vi "PV MiniTest Calibration.vi"(0 "VISA session":refnum<visa-resource-name>, 1 "Adress of unit":u16=1 min=1 max=999 step=1, 5 "Parameter":u16(ring) items=[" State of Calibration (read only)", " Calibration factor (read only)", " Start Calibration (write only)"], 11 "error in (no error)":errorcluster) -> (4 "dup VISA session":refnum<visa-resource-name>, 6 "response (data)":string, 15 "error out":errorcluster)   [LabVIEW 2021, in "Pfeiffer Vacuum.lvlib"]
doc: "There are 3 parameters available, only one of which can be enabled at a time. \n\n0 - Calibration State (default) - Para 667\n1 - Calibration factor (read only) - Para 696\n7 - Start Calibration (write only) - Para 699"
uses:
  <instrlib>/Pfeiffer Vacuum/Pfeiffer Vacuum.lvlib
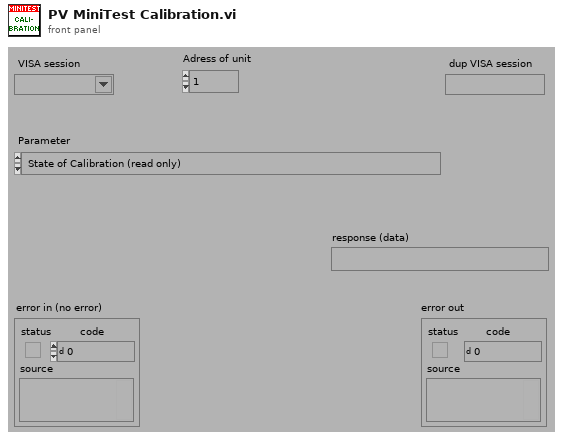
[diagram p1: front panel]
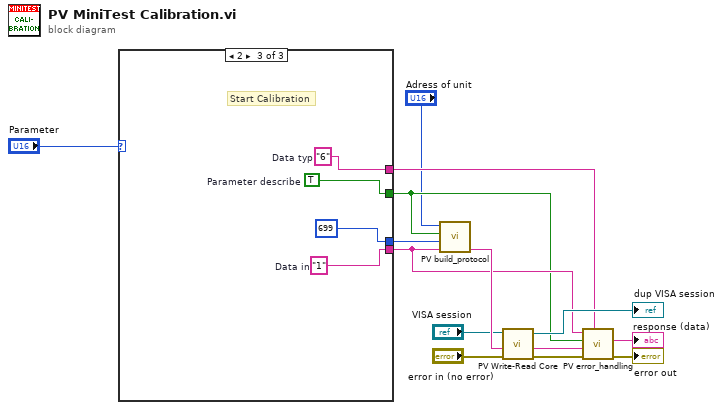
[diagram p0: block diagram]
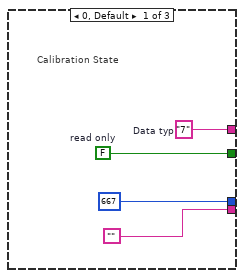
[diagram p2: hidden frame]
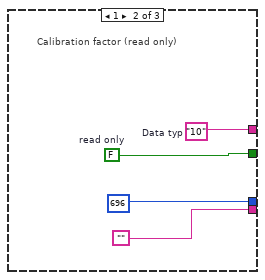
[diagram p3: hidden frame]
diagram:
  n1 = case shown="2" "Parameter" {
    tunnel: [u16 667 ("Parameter-number") u16 696 ("Parameter-number") u16 699 ("Parameter-number")] -> w14
    tunnel: ["" "" w23] -> w9
    tunnel: [w17 w22 w25] -> w7
    tunnel: [w18 w21 w26] -> w8
    frame 0, Default {
      w17 = FALSE  # read only
      w18 = "7"  # Data typ
      # "Calibration State"
    }
    frame 1 {
      w22 = FALSE  # read only
      w21 = "10"  # Data typ
      # "Calibration factor (read only)"
    }
    frame 2 {
      w23 = "1"  # Data in
      w25 = TRUE  # Parameter describe
      w26 = "6"  # Data typ
      # "Start Calibration"
    }
  }
  n2 = call <instrlib>:"PV build_protocol.vi"("Data"=w9, "Parameter-number"=w14, "parameter\nread<->describe"=w7, "Adress"="Adress of unit") -> ("output"=w13:string)  [unwired: 3 in]
  n3 = call <instrlib>:"PV Write-Read Core.vi"("error in"="error in (no error)", "Write data in"=w13, "VISA session"="VISA session") -> ("error out"=w11:errorcluster, "response (data) out"=w12:string, "dup VISA session"=→"dup VISA session":refnum<visa-resource-name>)  [unwired: 2 in]
  n4 = call <instrlib>:"PV error_handling.vi"("Data Typ in"=w8, "error in"=w11, "response (data) in"=w12, "Parameter\nread only<->describe"=w7, "data in"=w9) -> ("error out"=→"error out":errorcluster, "Data out"=→"response (data)":string)  [unwired: 4 in, 1 out]
